vi "set_delay.vi"(8 "error in (no error)":errorcluster {"code" format="%.0x"}, 10 "Delay":dbl, 11 "VISA Scope In":refnum<visa-resource-name>) -> (0 "error out":errorcluster {"code" format="%.0x"}, 3 "VISA Out":refnum<visa-resource-name>)   [LabVIEW 2011]
panel:
  out "Sent String":string
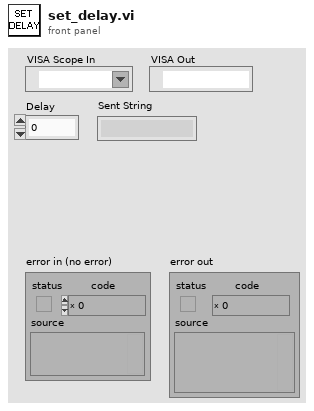
[diagram p1: front panel]
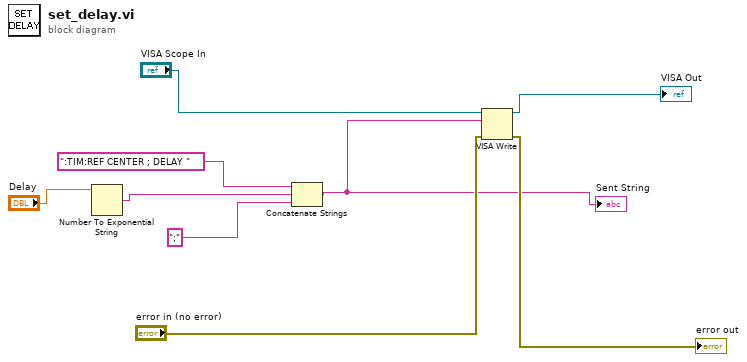
[diagram p0: block diagram]
diagram:
  n1 = Number To Exponential String(number="Delay") -> (E-format string=w2:string)  [unwired: 3 in]
  n2 = Concatenate Strings(":TIM:REF CENTER ; DELAY ", w2, ";" ("string")) -> (w5:string)
  "Sent String" <- w5
  n3 = VISA Write(VISA resource name="VISA Scope In", write buffer=w5, error in (no error)="error in (no error)") -> (VISA resource name out=→"VISA Out":refnum<visa-resource-name>, error out=→"error out":errorcluster)  [unwired: 1 out]
